vi "Actor Core.vi"(8 "error in":errorcluster, 11 "GObject View in":refnum<class "VI View.lvclass">) -> (0 "error out":errorcluster, 3 "Actor out":refnum<class "Actor.lvclass">)   [LabVIEW 2013, in "SET Project Editor.lvlib" / "VI View.lvclass"]
doc: "(<B>Filename</B>: Actor Framework.lvlib:Actor.lvclass:Actor Core.vi)\n\nReceives messages to the actor, reacts to them, and initiates any error handling that may shut the actor down.\n\nDescendant classes may override this VI to append parallel tasks for the actor to complete while it handles messages. Overrides use the Call Parent Method node."
uses:
  VI View.lvclass
  <vilib>/ActorFramework/Actor/Actor.lvclass
  <vilib>/ActorFramework/Actor/Actor.lvclass/Actor.ctl
  <vilib>/ActorFramework/Message Enqueuer/Message Enqueuer.lvclass/Message Enqueuer.ctl
  Controller Messages/Change Selection Msg/Change Selection Msg.lvclass/Change Selection Msg.ctl
  Controller Messages/Remove Object Msg/Remove Object Msg.lvclass/Remove Object Msg.ctl
  VI View.lvclass/VI View.ctl
  UI View/UI View.lvclass
  <vilib>/ActorFramework/Message Enqueuer/Init from Existing Queue.vi
  <vilib>/ActorFramework/Message Enqueuer/Enqueue.vi
  <vilib>/ActorFramework/Message Priority Queue/Priority Enqueue.vi
  <vilib>/ActorFramework/Message Enqueuer/Message Enqueuer.lvclass
  <vilib>/ActorFramework/Stop Msg/Stop Msg.lvclass
  Controller Messages/Change Selection Msg/Change Selection Msg.lvclass
  Controller Messages/Remove Object Msg/Remove Object Msg.lvclass
  UI View Messages/Preview Msg/Preview Msg.lvclass
panel:
  in  "Preview":bool
  out "Path":string
  in  "Items":i32(listbox)
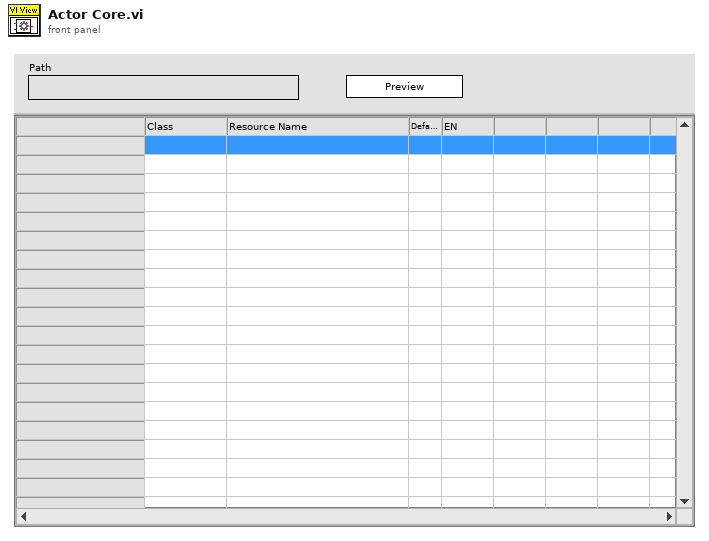
[diagram p1: front panel]
types:
  T1 = typedef "LVPoint32TypeDef.ctl" = cluster{"Horizontal":i32, "Vertical":i32}
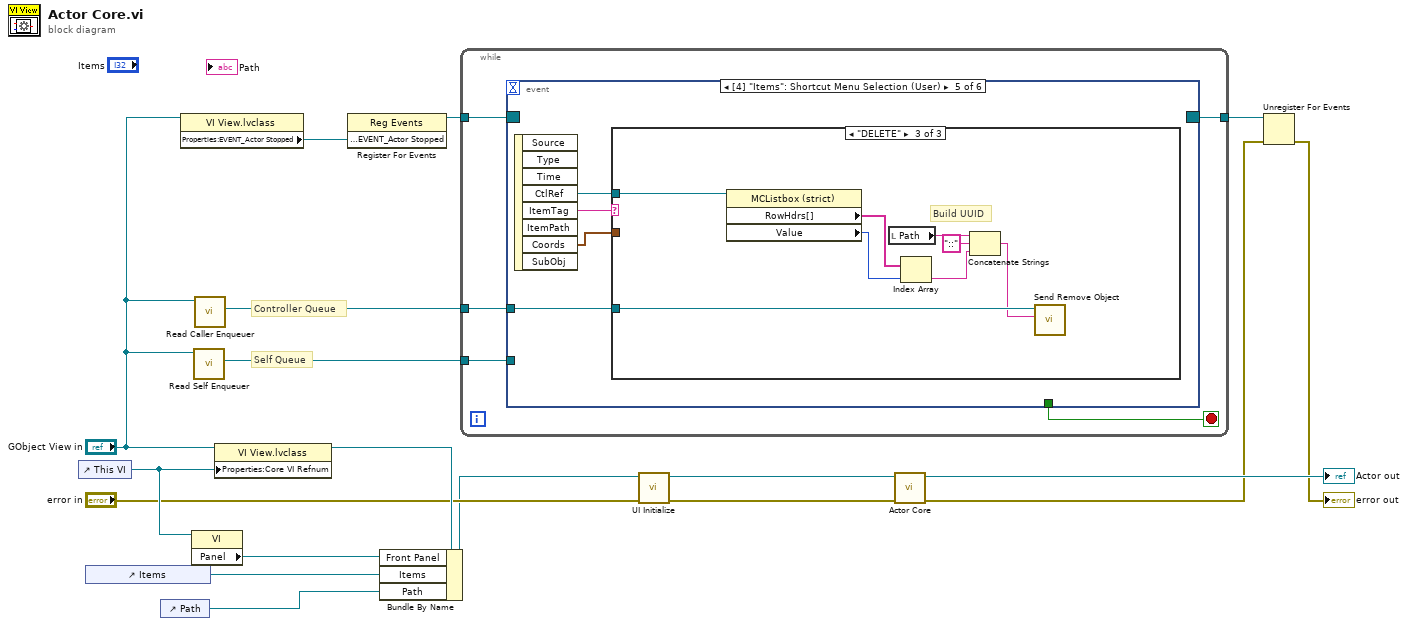
[diagram p0: block diagram]
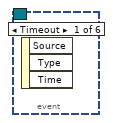
[diagram p2: hidden frame]
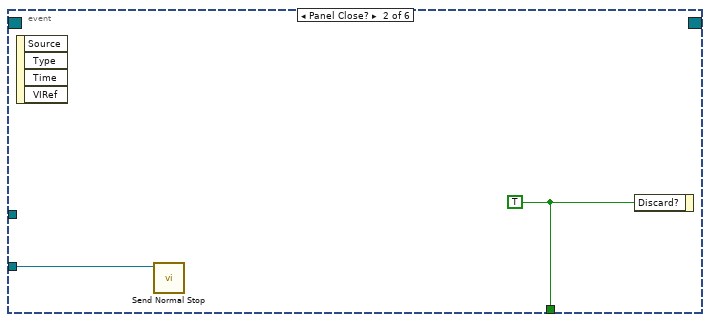
[diagram p3: hidden frame]
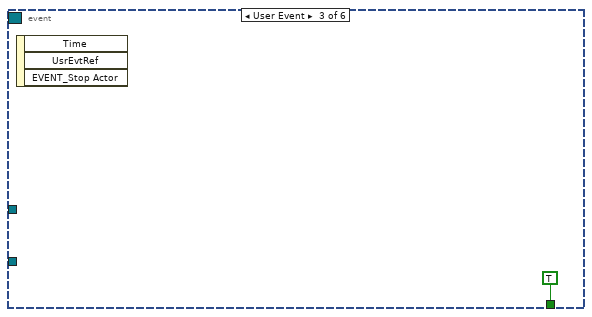
[diagram p4: hidden frame]
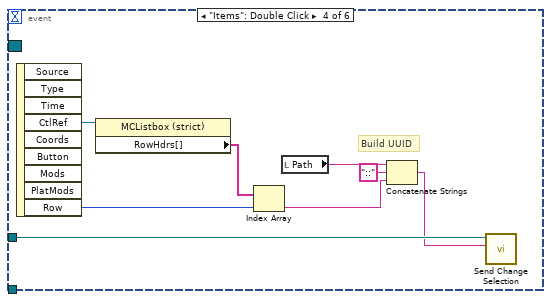
[diagram p5: hidden frame]
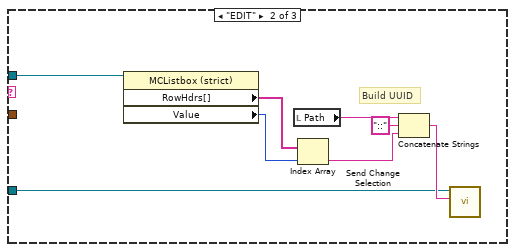
[diagram p7: hidden frame]
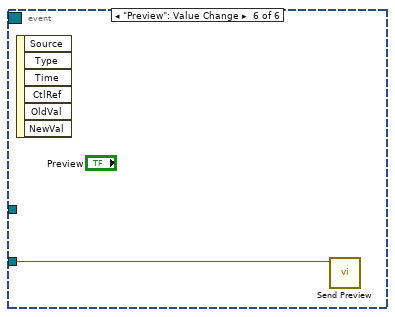
[diagram p8: hidden frame]
diagram:
  # "Controller Queue"
  # "Self Queue"
  n1 = control-ref of="This VI"() -> (w9:refnum<vi>)
  n2 = control-ref of="Items"() -> (w7:refnum<vi>)
  n3 = control-ref of="Path"() -> (w6:refnum<vi>)
  n4 = property class="VI View.lvclass"(reference="GObject View in") -> ("Properties:EVENT_Actor Stopped"=w17:refnum<user-event>)  [unwired: 1 in, 2 out]
  n5 = property class="VI"(reference=w9) -> ("Panel"=w8:refnum<vi>)  [unwired: 1 in, 2 out]
  n6 = call <vilib>:"Read Self Enqueuer.vi"("Actor"="GObject View in") -> ("Self Enqueuer"=w5:refnum<class "Message Enqueuer.lvclass">)  [unwired: 10 in]
  n7 = call <vilib>:"Read Caller Enqueuer.vi"("Actor"="GObject View in") -> ("Caller Enqueuer"=w12:refnum<class "Message Enqueuer.lvclass">)  [unwired: 10 in]
  n8 = property class="VI View.lvclass"(reference="GObject View in", "Properties:Core VI Refnum"=w9) -> (reference out=w10:refnum<class "VI View.lvclass">)  [unwired: 1 in, 1 out]
  n9 = register-events(w17) -> (reference out=w16:refnum<event-registration>)  [unwired: 2 in, 1 out]
  n10 = Bundle By Name(cluster=w10, "Front Panel"=w8, "Items"=w7, "Path"=w6) -> (w1:refnum<class "VI View.lvclass">)
  n11 = while {
    tunnel: w16 -> [w22]
    tunnel: [w21] -> w15
    tunnel: w5 -> [w20]
    tunnel: w12 -> [w19]
    stop <- w23 stop-if-true
    n12 = event shown="[4] \"Items\": Shortcut Menu Selection (User)" {
      selector: w22 -> [_ _ _ _ _ _]
      dyn-events: [_ _ _ _ _ _] -> w21
      timeout: _ -> [_ _ _ _ _ _]
      tunnel: [_ w25 TRUE ("Discard?") _ _ _] -> w23
      tunnel: w20 -> [_ w24 _ _ _ w55]
      tunnel: w19 -> [_ _ _ w28 w35 _]
      event Timeout {
        n13 = event-data() -> ()  [unwired: 1 in, 3 out]
      }
      event Panel Close? {
        w25 = TRUE ("Discard?")
        n14 = event-data() -> ()  [unwired: 1 in, 4 out]
        n15 = call <vilib>:"Send Normal Stop.vi"("Message Enqueuer"=w24) -> ()  [unwired: 10 in, 1 out]
        n16 = event-data("Discard?"=w25) -> ()  [unwired: 1 in, 1 out]
      }
      event User Event {
        n17 = event-data() -> ()  [unwired: 1 in, 3 out]
      }
      event "Items": Double Click {
        # "Build UUID"
        n18 = event-data() -> ("CtlRef"=w34:refnum<vi>, "Row"=w32:i32)  [unwired: 1 in, 7 out]
        n19 = property class="MCListbox (strict)"(reference=w34) -> ("RowHdrs[]"=w33:string[])  [unwired: 1 in, 2 out]
        n20 = Index Array(array=w33, index=w32) -> (element=w29:string)
        n21 = local read "Path"() -> (w31:string)
        n22 = Concatenate Strings(w31, "::" ("string"), w29) -> (w27:string)
        n23 = call "Send Change Selection.vi"("UID"=w27, "Message Enqueuer"=w28) -> ()  [unwired: 8 in, 2 out]
      }
      event "Items": Shortcut Menu Selection (User) {
        n24 = event-data() -> ("CtlRef"=w37:refnum<vi>, "ItemTag"=w38:string, "Coords"=w36:T1)  [unwired: 1 in, 5 out]
        n25 = case shown="\"DELETE\"" w38 {
          tunnel: w37 -> [_ w40 w49]
          tunnel: w36 -> [_ _ _]
          tunnel: w35 -> [_ w39 w48]
          frame Default {
          }
          frame "EDIT" {
            # "Build UUID"
            n26 = property class="MCListbox (strict)"(reference=w40) -> ("RowHdrs[]"=w45:string[], "Value"=w46:i32)  [unwired: 1 in, 2 out]
            n27 = local read "Path"() -> (w44:string)
            n28 = Index Array(array=w45, index=w46) -> (element=w42:string)
            n29 = Concatenate Strings(w44, "::" ("string"), w42) -> (w41:string)
            n30 = call "Send Change Selection.vi"("UID"=w41, "Message Enqueuer"=w39) -> ()  [unwired: 8 in, 2 out]
          }
          frame "DELETE" {
            # "Build UUID"
            n31 = property class="MCListbox (strict)"(reference=w49) -> ("RowHdrs[]"=w53:string[], "Value"=w54:i32)  [unwired: 1 in, 2 out]
            n32 = local read "Path"() -> (w52:string)
            n33 = Index Array(array=w53, index=w54) -> (element=w50:string)
            n34 = Concatenate Strings(w52, "::" ("string"), w50) -> (w47:string)
            n35 = call "Send Remove Object.vi"("UUID"=w47, "Message Enqueuer"=w48) -> ()  [unwired: 8 in, 2 out]
          }
        }
      }
      event "Preview": Value Change {
        n36 = event-data() -> ()  [unwired: 1 in, 6 out]
        n37 = call "Send Preview.vi"("Message Enqueuer"=w55) -> ()  [unwired: 9 in, 2 out]
      }
    }
  }
  n38 = call-dynamic "UI Initialize.vi"("error in (no error)"="error in", "GObject View in"=w1) -> ("error out"=w3:errorcluster, "GObject View out"=w4:refnum<class "VI View.lvclass">)  [unwired: 8 in]
  n39 = call-parent "Actor Core.vi"("error in"=w3, "Actor in"=w4) -> ("error out"=w14:errorcluster, "Actor out"=→"Actor out":refnum<class "Actor.lvclass">)  [unwired: 8 in]
  n40 = Unregister For Events(event registration refnum=w15, error in=w14) -> (error out=→"error out":errorcluster)
